vi "tcp_demonstration.vi"() -> ()   [LabVIEW 2018]
panel:
  in  "stop":bool
  out "data out":string
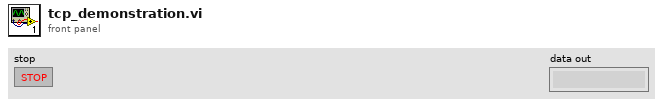
[diagram p1: front panel]
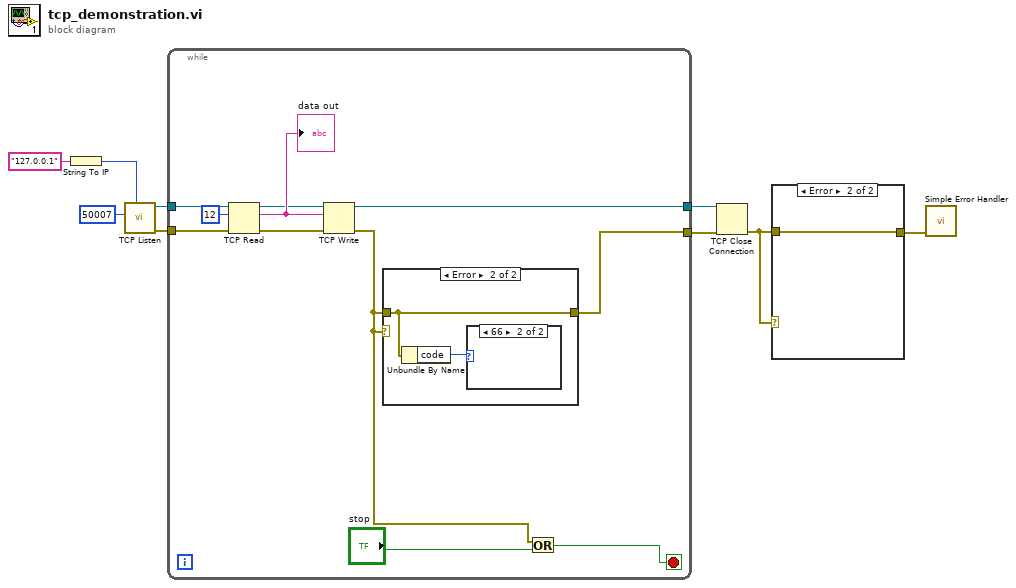
[diagram p0: block diagram]
diagram:
  n1 = String To IP(1:"127.0.0.1" ("name")) -> (0:w8:u32)
  n2 = call <vilib>:"TCP Listen.vi"("net address"=w8, "port"=u16 50007) -> ("error out"=w5:errorcluster, "connection ID"=w6:refnum<k5>)  [unwired: 5 in, 3 out]
  n3 = while {
    tunnel: w6 -> [w19]
    tunnel: w5 -> [w20]
    tunnel: [w12] -> w4
    tunnel: [w11] -> w3
    stop <- w14 stop-if-true
    n4 = TCP Read(connection ID=w19, bytes to read=12, error in (no error)=w20) -> (connection ID out=w15:refnum<k5>, data out=w17:string, error out=w16:errorcluster)  [unwired: 2 in]
    "data out" <- w17
    n5 = TCP Write(connection ID=w15, data in=w17, error in (no error)=w16) -> (connection ID out=w11:refnum<k5>, error out=w10:errorcluster)  [unwired: 1 in, 1 out]
    n6 = case shown="Error" w10 {
      tunnel: [w21 w23] -> w12
      tunnel: w10 -> [w21 w23]
      frame No Error {
      }
      frame Error {
        n7 = Unbundle By Name(w23) -> ("code"=w22:i32)
        n8 = case shown="66" w22 {
          frame 0, Default {
          }
          frame 66 {
          }
        }
      }
    }
    n9 = Or(x=w10, y="stop") -> (x .or. y?=w14:bool)
  }
  n10 = TCP Close Connection(connection ID=w3, error in (no error)=w4) -> (error out=w2:errorcluster)  [unwired: 1 in, 1 out]
  n11 = case shown="Error" w2 {
    tunnel: [w24 w25] -> w1
    tunnel: w2 -> [w24 w25]
    frame No Error {
    }
    frame Error {
    }
  }
  n12 = call <vilib>:"Simple Error Handler.vi"("error in (no error)"=w1) -> ()  [unwired: 4 in, 5 out]
